vi "PID_Xaxis_sandbox.vi"() -> ()   [LabVIEW 2019]
uses:
  <vilib>/myRIO/Common/Instrument Driver Framework/myRIO v1.0/UART/vis/myRIO v1.0 Close UART.vi
  <vilib>/addons/control/pid/pid.llb/PID (DBL).vi
  <vilib>/myRIO/Common/Instrument Driver Framework/Utilities/vis/FPGA Ref Manager.vi
  <vilib>/myRIO/Common/Instrument Driver Framework/myRIO v1.0/myRIO v1.0 Reset FPGA.vi
  <vilib>/myRIO/Common/Instrument Driver Framework/myRIO v1.0/IRQ/vis/myRIO v1.0 IRQ Info FGV.vi
  <vilib>/myRIO/Common/Instrument Driver Framework/myRIO v1.0/IRQ/vis/myRIO v1.0 Timer IRQ Info FGV.vi
  <vilib>/myRIO/Common/Instrument Driver Framework/myRIO v1.0/IRQ/vis/myRIO v1.0 ISR Agent.vi
  <vilib>/myRIO/Instrument Drivers/Utilities/vis/Reset Index.vi
  <vilib>/myRIO/Common/Instrument Driver Framework/myRIO v1.0/Resource Manager/vis/myRIO v1.0 Block Write Resource Manager.vi
  <vilib>/addons/control/pid/NI_PID_pid.lvlib
  <vilib>/myRIO/Instrument Drivers/Utilities/Utilities.lvlib
panel:
  in  "error in (no error)":errorcluster
  out "error out":errorcluster
  out "PID Out":dbl=1.8829840965238862 format="%0#4.1g"
  in  "Reinitialize":bool
  in  "PID Gains":T1={"Proportional Gain (Kc)"=0.8, "Integral Gain"=25.0, "Derivative Gain"=0.004}
  in  "stop":bool
  in  "X In":dbl format="%#_13g"
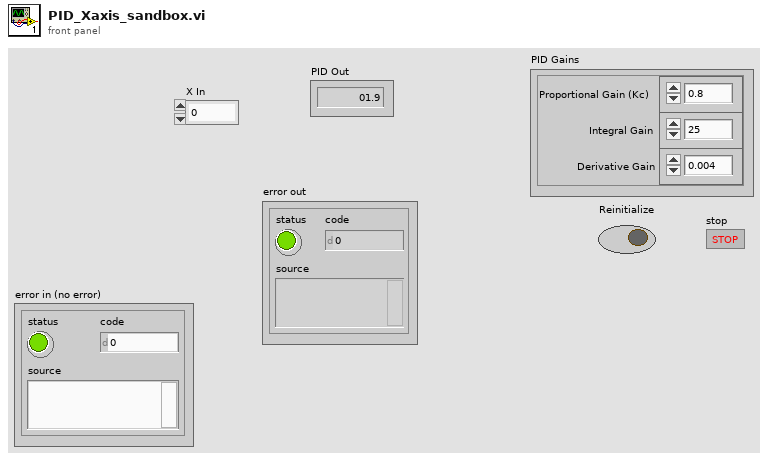
[diagram p1: front panel]
types:
  T1 = cluster{"Proportional Gain (Kc)":dbl, "Integral Gain":dbl, "Derivative Gain":dbl}
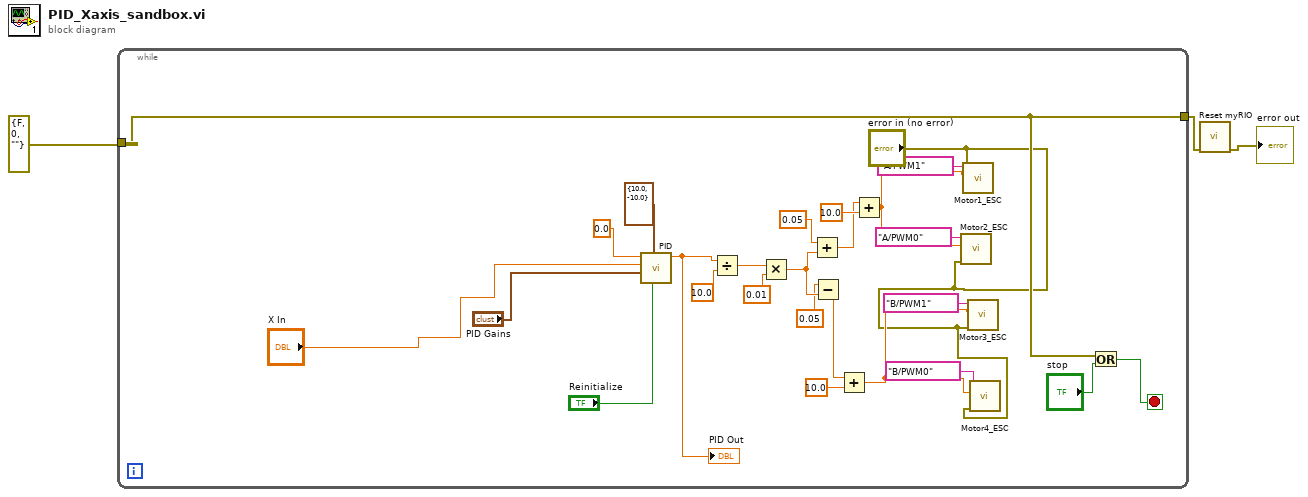
[diagram p0: block diagram]
diagram:
  n1 = while {
    tunnel: errorcluster {"status"=FALSE, "code"=0, "source"=""} ("error in (no error)") -> [w16]
    tunnel: [w16] -> w1
    stop <- w17 stop-if-true
    n2 = call-poly <vilib>:"PID.vi"("reinitialize? (F)"="Reinitialize", "output range"=cluster{"output high":dbl, "output low":dbl} {"output high"=10.0, "output low"=-10.0}, "PID gains"="PID Gains", "process variable"="X In", "setpoint"=0.0 ("Angle (rads)")) -> ("output"=w21:dbl)  [unwired: 5 in, 1 out]
    "PID Out" <- w21
    n3 = Divide(x=w21, y=10.0) -> (x/y=w28:dbl)
    n4 = Multiply(x=w28, y=0.01) -> (x*y=w27:dbl)
    n5 = Add(x=0.05, y=w27) -> (x+y=w11:dbl)
    n6 = Subtract(x=0.05, y=w27) -> (x-y=w12:dbl)
    n7 = Add(x=w12, y=10.0) -> (x+y=w9:dbl)
    n8 = Add(x=w11, y=10.0) -> (x+y=w10:dbl)
    n9 = call "Motor2_ESC.vi"("error in (no error)"="error in (no error)", "Percent Power"=w10, "Channel Name"=tag "A/PWM0") -> ()  [unwired: 8 in, 1 out]
    n10 = call "Motor1_ESC.vi"("error in (no error)"="error in (no error)", "Percent Power"=w10, "Channel Name"=tag "A/PWM1") -> ()  [unwired: 8 in, 1 out]
    n11 = call "Motor3_ESC.vi"("error in (no error)"="error in (no error)", "Percent Power"=w9, "Channel Name"=tag "B/PWM1") -> ()  [unwired: 8 in, 1 out]
    n12 = call "Motor4_ESC.vi"("error in (no error)"="error in (no error)", "Percent Power"=w9, "Channel Name"=tag "B/PWM0") -> ()  [unwired: 8 in, 1 out]
    n13 = Or(x=w16, y="stop") -> (x .or. y?=w17:bool)
  }
  n14 = call <vilib>:"Reset myRIO.vi"("error in (no error)"=w1) -> ("error out"=→"error out":errorcluster)  [unwired: 10 in]
